vi "Get SMO PGSQL Log Paths.vi"(8 "error in (no error)":errorcluster, 11 "instrument.PPMS in":refnum<class "instrument.PPMS.lvclass">) -> (0 "error out":errorcluster, 2 "Paths":string, 3 "instrument.PPMS out":refnum<class "instrument.PPMS.lvclass">)   [LabVIEW 2019, in "instrument.PPMS.lvclass"]
uses:
  instrument.PPMS.lvclass
  <userlib>/LevyLab/Instrument Framework/Instrument Types/Cryostat/Instrument.Cryostat.lvclass
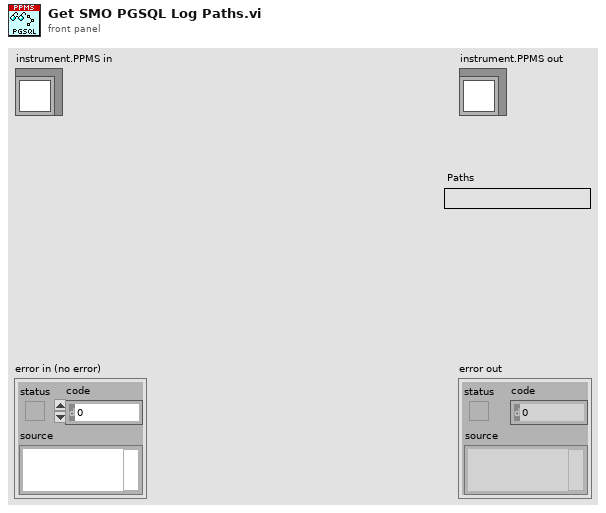
[diagram p1: front panel]
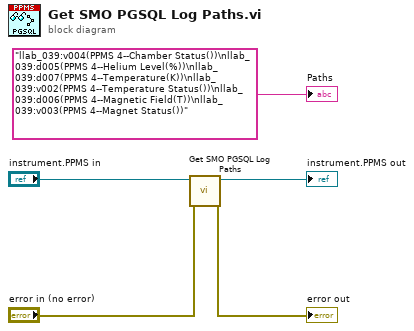
[diagram p0: block diagram]
diagram:
  n1 = call-parent "Get SMO PGSQL Log Paths.vi"("error in (no error)"="error in (no error)", "Instrument in"="instrument.PPMS in") -> ("error out"=→"error out":errorcluster, "Instrument out"=→"instrument.PPMS out":refnum<class "instrument.PPMS.lvclass">)  [unwired: 7 in, 1 out]
  "Paths" <- "llab_039:v004(PPMS 4--Chamber Status())\nllab_039:d005(PPMS 4--Helium Level(%))\nllab_039:d007(PPMS 4--Temperature(K))\nllab_039:v002(PPMS 4--Temperature Status())\nllab_039:d006(PPMS 4--Magnetic Field(T))\nllab_039:v003(PPMS 4--Magnet Status())" ("Paths")
